vi "act_solenoids.vi"   [LabVIEW 2018]
uses:
  <vilib>/rvi/DataTransferAndStorage/Container/Common/niFpgaContainerExecOnDevCompGetState.vi
  <vilib>/rvi/Emulation/niFpgaEmulationIsFPGAContextNoSignature.vi
  <vilib>/rvi/DataTransferAndStorage/Container/Common/niFpgaContainerGetUniqueNameForEmu.vi
  <vilib>/rvi/Memory/Memory_Emulation/niFpgaMemoryEmulationCacheClearOnFirstRun.vi
  <vilib>/rvi/Memory/Memory_Emulation/nirvimemoryEmulationManagerCache_MakeExclusive.vi
  <vilib>/rvi/Memory/Memory_Emulation/niFpgaMemoryEmulationValidateCache.vi
  <vilib>/rvi/Memory/Memory_Emulation/nirvimemoryEmulationManagerCache_InsertValue.vi
  <vilib>/Utility/error.llb/Clear Errors.vi
  <vilib>/rvi/Memory/Memory_Emulation/nirvimemoryEmulationManagerCache_ReleaseExclusive.vi
  <vilib>/rvi/Memory/Memory_Emulation/nirvimemoryEmulationManagerCache_GetValue.vi
  <vilib>/rvi/Memory/Memory_Emulation/nirvimemoryEmulationManagerCache_SetValue.vi
  <vilib>/rvi/Emulation/niFpgaProcessEmulError.vi
  <vilib>/rvi/Emulation/niFpgaSctlEmulationGetInTimedLoop.vi
  <vilib>/rvi/eio/common/nirviEmuTemplateMethod_errors.vi
  <vilib>/rvi/DataTransferAndStorage/Container/XNode/niFpgaContainer.xnode
  <vilib>/rvi/DataTransferAndStorage/Register/Emulation/niFpgaRegisterEmulationRefIn.vi
  <vilib>/eio/EIONode/EIONode.xnode
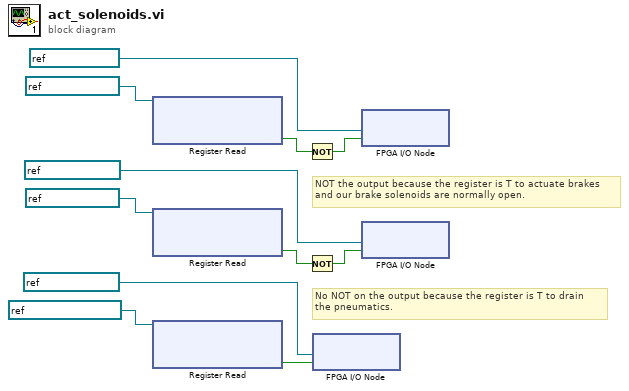
[diagram p0: block diagram]
diagram:
  # "No NOT on the output because the register is T to drain\nthe pneumatics."
  # "NOT the output because the register is T to actuate brakes\nand our brake solenoids are normally open."
  n1 = xnode "Register Read"("Register In"=refnum<k21> "REG_brake_1") -> ("Data"=w9:bool)  [unwired: 1 out]
  n2 = xnode "Register Read"("Register In"=refnum<k21> "REG_brake_2") -> ("Data"=w6:bool)  [unwired: 1 out]
  n3 = xnode "Register Read"("Register In"=refnum<k21> "REG_drain_valve") -> ("Data"=w3:bool)  [unwired: 1 out]
  n4 = Not(x=w9) -> (.not. x?=w2:bool)
  n5 = Not(x=w6) -> (.not. x?=w1:bool)
  n6 = xnode "FPGA I/O Node"("I/O Item"=w3, "FPGA I/O In"=refnum<k21> "Mod2/DIO11") -> ()  [unwired: 1 out]
  n7 = xnode "FPGA I/O Node"("I/O Item"=w2, "FPGA I/O In"=refnum<k21> "Mod2/DIO9") -> ()  [unwired: 1 out]
  n8 = xnode "FPGA I/O Node"("I/O Item"=w1, "FPGA I/O In"=refnum<k21> "Mod2/DIO10") -> ()  [unwired: 1 out]
